vi "Draw Tangent Circle.vi"(10 "Cluster":cluster{dbl, dbl}, 11 "Numeric":dbl) -> (3 "Array":cluster{dbl, dbl}[](array[cluster]))   [LabVIEW 2019]
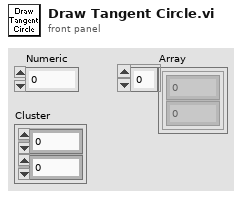
[diagram p1: front panel]
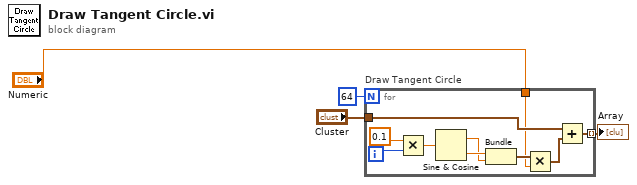
[diagram p0: block diagram]
diagram:
  n1 = for "Draw Tangent Circle" {
    N: 64 -> [_]
    tunnel: "Cluster" -> [w9]
    tunnel: [w8] -> w3 mode=indexing
    tunnel: "Numeric" -> [w5]
    i -> [w14]
    n2 = Multiply(x=0.1, y=w14) -> (x*y=w12:dbl)
    n3 = Sine & Cosine(0:w12) -> (1:w10:dbl, 2:w11:dbl)
    n4 = Bundle(w11, w10) -> (w7:cluster{dbl, dbl})  [unwired: 1 in]
    n5 = Multiply(x=w7, y=w5) -> (x*y=w6:cluster{dbl, dbl})
    n6 = Add(x=w9, y=w6) -> (x+y=w8:cluster{dbl, dbl})
  }
  "Array" <- w3
